vi "Read isAlive.vi"(8 "error in (no error)":errorcluster, 11 "MotorController in":refnum<class "MotorController.lvclass">) -> (0 "error out":errorcluster, 2 "isAlive":bool, 3 "MotorController out":refnum<class "MotorController.lvclass">)   [LabVIEW 2017, in "MotorController.lvclass"]
uses:
  MotorController.lvclass
  MotorController.lvclass/MotorController.ctl
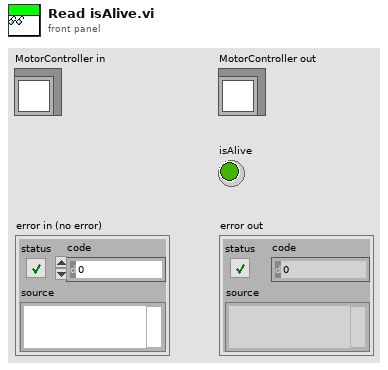
[diagram p1: front panel]
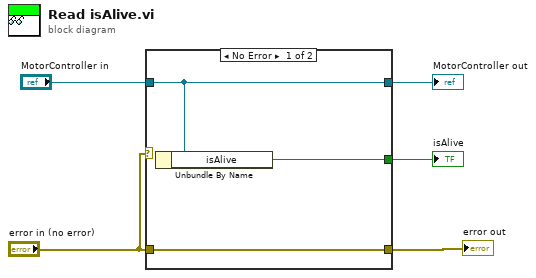
[diagram p0: block diagram]
diagram:
  n1 = case shown="No Error" "error in (no error)" {
    tunnel: "MotorController in" -> [w6 w9]
    tunnel: [w8 _] -> w4
    tunnel: [w7 w10] -> w3
    tunnel: "error in (no error)" -> [w7 w10]
    tunnel: [w6 w9] -> w1
    frame No Error {
      n2 = Unbundle By Name(w6) -> ("isAlive"=w8:bool)
    }
    frame Error {
    }
  }
  "MotorController out" <- w1
  "isAlive" <- w4
  "error out" <- w3
